vi "DrawSpaceship_Intensity.vi"(9 "InitCluster_IN":T2) -> (1 "InitCluster_OUT":T2, 3 "spaceship_position":T1)   [LabVIEW 2022 SP3]
uses:
  InitCluster.ctl
  CharacterCluster.ctl
  <vilib>/picture/picture.llb/imagedata.ctl
  ShotInitCluster.ctl
  <vilib>/Utility/miscctls.llb/LVPositionTypeDef.ctl
  <vilib>/Utility/miscctls.llb/LVBoundsTypeDef.ctl
  ShotCluster.ctl
  move_dir_ud.ctl
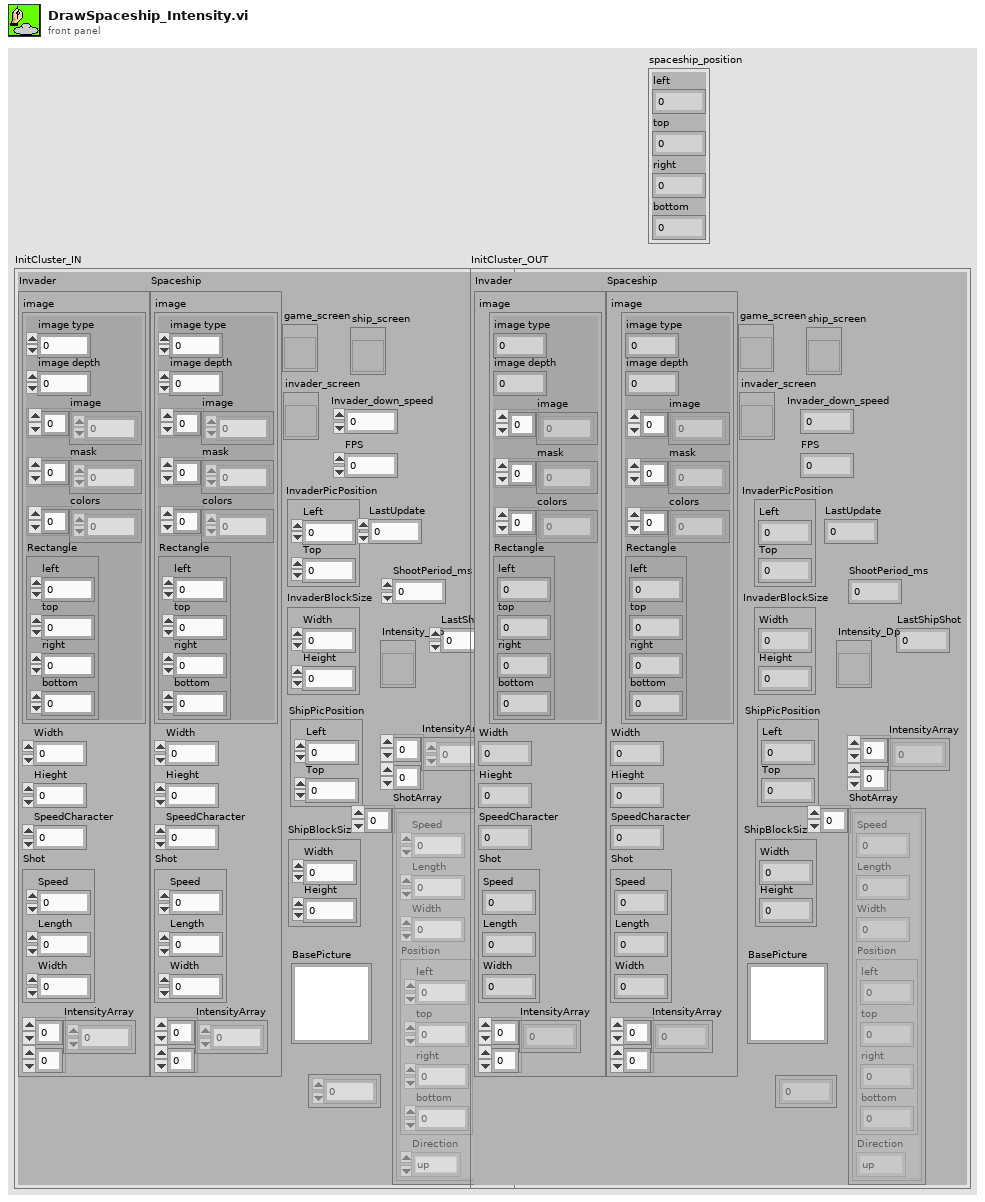
[diagram p1: front panel]
types:
  T1 = cluster{"left":i16, "top":i16, "right":i16, "bottom":i16}
  T2 = typedef "InitCluster.ctl" = cluster{"Invader":T3, "Spaceship":T3, "game_screen":refnum<vi>, "BasePicture":picture, "invader_screen":refnum<vi>, "InvaderPicPosition":T6, "Invader_down_speed":i16, "FPS":u16, "InvaderBlockSize":T7, "ship_screen":refnum<vi>, "ShipBlockSize":T7, "ShipPicPosition":T6, "LastUpdate":u32, "Intensity_Dp":refnum<vi>, "IntensityArray":u8[][], "ShotArray":T8[], "InvaderShotTimeArray":u32[], "ShootPeriod_ms":i32, "LastShipShot":u32}
  T3 = typedef "CharacterCluster.ctl" = cluster{"image":T4, "Width":u32, "Hieght":u32, "SpeedCharacter":u32, "Shot":T5, "IntensityArray":u8[][]}
  T4 = typedef "imagedata.ctl" = cluster{"image type":i32, "image depth":i32, "image":u8[], "mask":u8[], "colors":u32[], "Rectangle":cluster{"left":i16, "top":i16, "right":i16, "bottom":i16}}
  T5 = typedef "ShotInitCluster.ctl" = cluster{"Speed":u32, "Length":u32, "Width":u32}
  T6 = typedef "LVPositionTypeDef.ctl" = cluster{"Left":i32, "Top":i32}
  T7 = typedef "LVBoundsTypeDef.ctl" = cluster{"Width":u32, "Height":u32}
  T8 = typedef "ShotCluster.ctl" = cluster{"Speed":u32, "Length":u32, "Width":u32, "Position":cluster{"left":i16, "top":i16, "right":i16, "bottom":i16}, "Direction":T9}
  T9 = typedef "move_dir_ud.ctl" = enum16{"up", "down"}
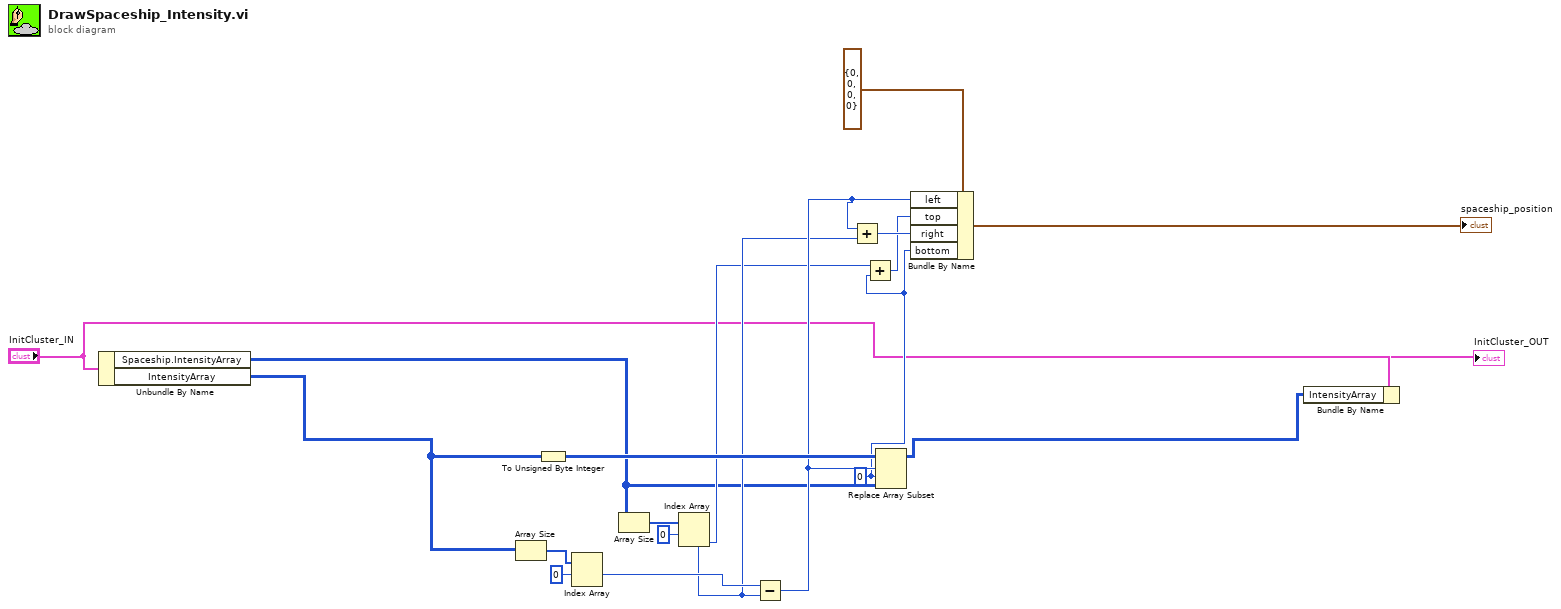
[diagram p0: block diagram]
diagram:
  w9 = 0 ("disabled index (col)")
  n1 = Unbundle By Name("InitCluster_IN") -> ("Spaceship.IntensityArray"=w5:u8[][], "IntensityArray"=w4:u8[][])
  n2 = Array Size(array=w4) -> (size(s)=w16:i32[])
  n3 = To Unsigned Byte Integer(number=w4) -> (unsigned 8bit integer=w19:u8[][])
  n4 = Index Array(array=w16, index #1=0 ("index")) -> (element #1=w14:i32)  [unwired: 1 in, 1 out]
  n5 = Array Size(array=w5) -> (size(s)=w18:i32[])
  n6 = Index Array(array=w18, index #1=0 ("index")) -> (element #1=w11:i32, element #2=w8:i32)  [unwired: 1 in]
  n7 = Subtract(x=w14, y=w11) -> (x-y=w12:i32)
  n8 = Add(x=w12, y=w11) -> (x+y=w10:i32)
  n9 = Add(x=w8, y=w9) -> (x+y=w7:i32)
  n10 = Replace Array Subset(array=w19, new element=w5, index (row)=w12, index (col)=w9) -> (w1:u8[][])
  n11 = Bundle By Name(cluster=T1 {"left"=0, "top"=0, "right"=0, "bottom"=0} ("SpaceshipPosition"), "left"=w12, "top"=w7, "right"=w10, "bottom"=w9) -> (→"spaceship_position":T1)
  n12 = Bundle By Name(cluster="InitCluster_IN", "IntensityArray"=w1) -> (→"InitCluster_OUT":T2)
